vi "Get Template Path.vi"(11 "Message Maker in":refnum<class "Message Scripter.lvclass">) -> (2 "Template Path":path)   [LabVIEW 2020, in "Message Maker.lvlib" / "Message Scripter.lvclass"]
uses:
  Message Scripter.lvclass
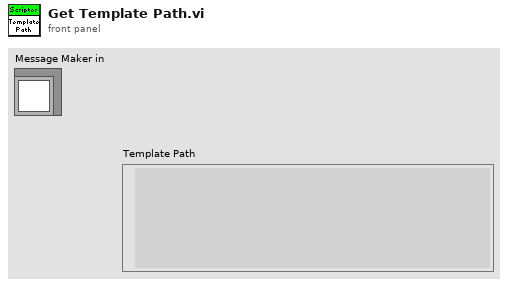
[diagram p1: front panel]
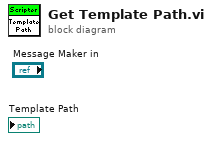
[diagram p0: block diagram]
diagram:
